vi "tt20_make_histogram.vi"(8 "error in (no error)":errorcluster, 10 "histo_settings":T1, 11 "tt20 in":refnum<class "tt20.lvclass">) -> (0 "error out":errorcluster, 3 "tt20 out":refnum<class "tt20.lvclass">)   [LabVIEW 2015, in "tt20.lvclass"]
uses:
  tt20.lvclass
  tt20_histo_settings_tdef.ctl
  tt20.lvclass/tt20.ctl
  C:/Users/MX-Microscope/Documents/LabVIEW Data/lvoop_campus_2018/Detector_Class/Swabian/time_tagger_vis/TTCSharp32.dll
  time_tagger_vis/TTCSharp32.dll
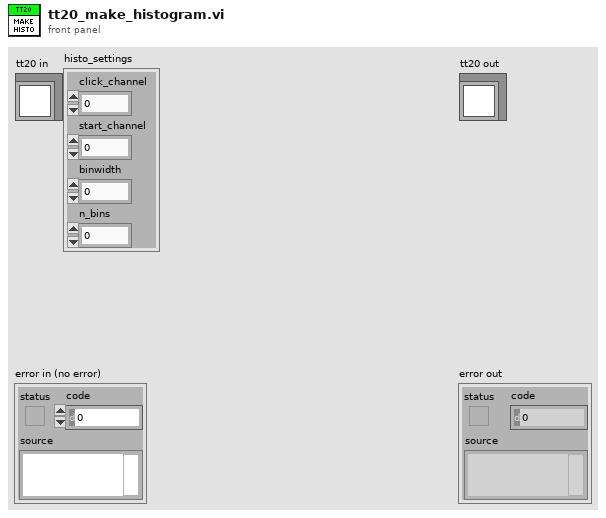
[diagram p1: front panel]
types:
  T1 = typedef "tt20_histo_settings_tdef.ctl" = cluster{"click_channel":u32, "start_channel":u32, "binwidth":i64, "n_bins":i32}
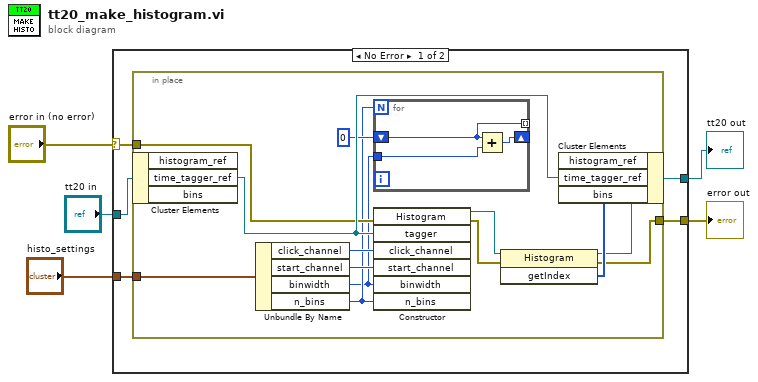
[diagram p0: block diagram]
diagram:
  n1 = case shown="No Error" "error in (no error)" {
    selector: "error in (no error)" -> [w10 w28]
    tunnel: [w9 w28] -> w4
    tunnel: [w6 w27] -> w2
    tunnel: "tt20 in" -> [w7 w27]
    tunnel: "histo_settings" -> [w8 _]
    frame No Error {
      n2 = in-place {
        in-place-border: w10 -> [w22]
        in-place-border: [w11] -> w9
        in-place-border: w8 -> [w21]
        n3 = in-place-cluster #1(w7) -> ("time_tagger_ref"=w23:refnum<k24>)  [unwired: 2 out]
        n4 = Unbundle By Name(w21) -> ("click_channel"=w20:u32, "start_channel"=w19:u32, "binwidth"=w16:i64, "n_bins"=w17:i32)
        n5 = for {
          N: w17 -> [_]
          tunnel: w16 -> [w26]
          tunnel: [w25] -> _ mode=indexing
          shift-right: [w24] -> _
          shift-left: 0 -> [w25]
          n6 = Add(x=w25, y=w26) -> (x+y=w24:i64)
        }
        n7 = constructor class="Histogram"(error in=w22, "tagger"=w23, "click_channel"=w20, "start_channel"=w19, "binwidth"=w16, "n_bins"=w17) -> (reference out=w15:refnum<k24>, error out=w12:errorcluster)  [unwired: 2 in, 6 out]
        n8 = invoke class="Histogram" method="getIndex"(reference=w15, error in=w12) -> (reference out=w13:refnum<k24>, error out=w11:errorcluster, "getIndex"=w14:i64[])  [unwired: 1 in]
        n9 = in-place-cluster #1("histogram_ref"=w13, "time_tagger_ref"=w23, "bins"=w14) -> (w6:refnum<class "tt20.lvclass">)
      }
    }
    frame Error {
    }
  }
  "error out" <- w4
  "tt20 out" <- w2
